vi "FPP-sample-download.vi"() -> ()   [LabVIEW 2016]
panel:
  in  "file path":path
  out "Vp2":dbl[](array[numeric]) format="%.2f"
  out "Time":dbl[](array[numeric]) format="%.2f"
  out "Vp1":dbl[](array[numeric]) format="%.2f"
  out "Id":dbl[](array[numeric]) format="%.2f"
  out "Ig":dbl[](array[numeric]) format="%.2f"
  out "error out":errorcluster
  out "VISA Resource Name out":refnum<visa-resource-name>
  in  "error in (no error)":errorcluster
  in  "VISA resource name in":refnum<visa-resource-name>
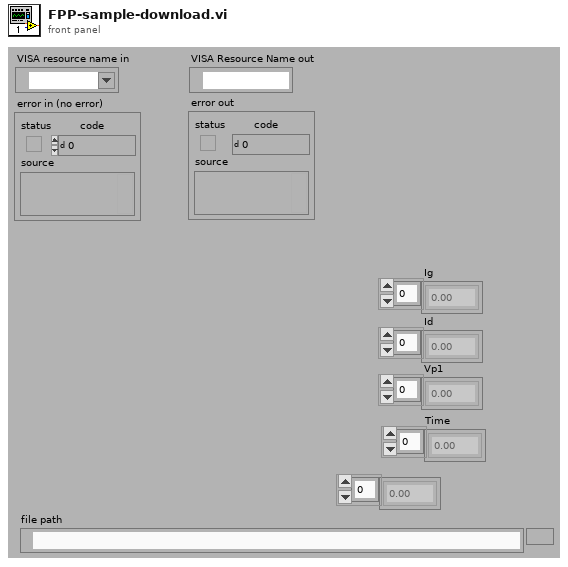
[diagram p1: front panel]
types:
  T1 = enum16{"open", "replace", "create", "open or create", "replace or create", "replace or create with confirmation"}
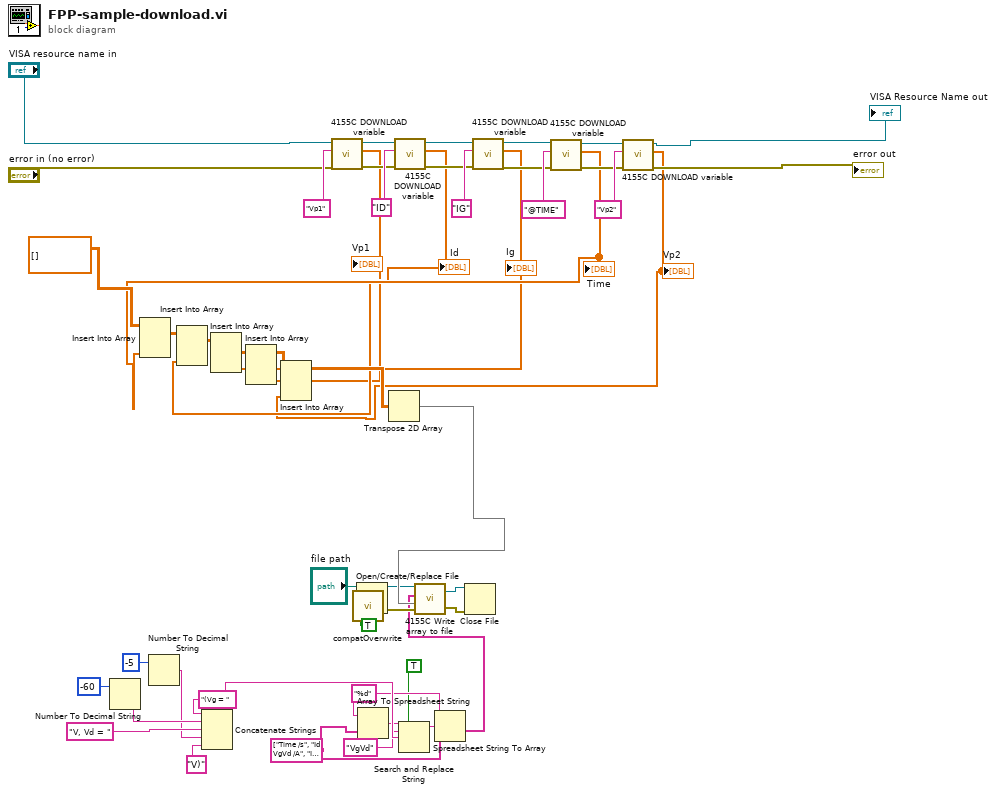
[diagram p0: block diagram]
diagram:
  w12 = string[] ["Time /s", "Id VgVd /A", "Ig VgVd /A", "Vp1 VgVd /V", "Vp2 VgVd /V"] ("Header")
  w16 = "%d" ("format string")
  n1 = Number To Decimal String(number=-60) -> (decimal integer string=w28:string)  [unwired: 1 in]
  n2 = Number To Decimal String(number=-5) -> (decimal integer string=w26:string)  [unwired: 1 in]
  n3 = Concatenate Strings("(Vg = " ("Substring"), w28, "V, Vd = " ("Substring"), w26, "V)" ("Substring")) -> (w24:string)
  n4 = call "4155C DOWNLOAD variable.vi"("error in (no error)"="error in (no error)", "Variable name"="Vp1", "VISA resource name in"="VISA resource name in") -> ("error out"=w49:errorcluster, "Output data"=w3:dbl[], "VISA Resource Name out"=w48:refnum<visa-resource-name>)  [unwired: 2 in]
  "Vp1" <- w3
  n5 = call <vilib>:"compatOverwrite.vi"("overwrite (F)"=TRUE) -> ("overwrite?"=w1:T1)
  n6 = Open/Create/Replace File(file path (use dialog)="file path", operation (0:open)=w1) -> (refnum out=w21:refnum<file>, error out=w22:errorcluster)  [unwired: 4 in, 1 out]
  n7 = Array To Spreadsheet String(array=w12, 3:w16) -> (spreadsheet string=w18:string)  [unwired: 1 in]
  n8 = call "4155C DOWNLOAD variable.vi"("error in (no error)"=w49, "Variable name"="ID", "VISA resource name in"=w48) -> ("error out"=w46:errorcluster, "Output data"=w5:dbl[], "VISA Resource Name out"=w45:refnum<visa-resource-name>)  [unwired: 2 in]
  "Id" <- w5
  n9 = Search and Replace String(replace all?=TRUE ("replace all? (F)"), input string=w18, search string="VgVd", replace string=w24) -> (result string=w14:string)  [unwired: 4 in, 3 out]
  n10 = Spreadsheet String To Array(format string=w16, spreadsheet string=w14, array type (2D Dbl)=w12) -> (array=w13:string[])  [unwired: 1 in]
  n11 = call "4155C DOWNLOAD variable.vi"("error in (no error)"=w46, "Variable name"="IG", "VISA resource name in"=w45) -> ("error out"=w42:errorcluster, "Output data"=w4:dbl[], "VISA Resource Name out"=w43:refnum<visa-resource-name>)  [unwired: 2 in]
  "Ig" <- w4
  n12 = call "4155C DOWNLOAD variable.vi"("error in (no error)"=w42, "Variable name"="@TIME", "VISA resource name in"=w43) -> ("error out"=w39:errorcluster, "Output data"=w6:dbl[], "VISA Resource Name out"=w40:refnum<visa-resource-name>)  [unwired: 2 in]
  "Time" <- w6
  n13 = Insert Into Array(array=dbl[][] [] ("Input Array"), new element=w6) -> (w34:dbl[][])  [unwired: 2 in]
  n14 = Insert Into Array(array=w34, new element=w5) -> (w33:dbl[][])  [unwired: 2 in]
  n15 = Insert Into Array(array=w33, new element=w4) -> (w32:dbl[][])  [unwired: 2 in]
  n16 = Insert Into Array(array=w32, new element=w3) -> (w31:dbl[][])  [unwired: 2 in]
  n17 = call "4155C DOWNLOAD variable.vi"("error in (no error)"=w39, "Variable name"="Vp2", "VISA resource name in"=w40) -> ("error out"=→"error out":errorcluster, "Output data"=w2:dbl[], "VISA Resource Name out"=→"VISA Resource Name out":refnum<visa-resource-name>)  [unwired: 2 in]
  "Vp2" <- w2
  n18 = Insert Into Array(array=w31, new element=w2) -> (w11:dbl[][])  [unwired: 2 in]
  n19 = Transpose 2D Array(2D array=w11) -> (transposed array=w30:dbl[][])
  n20 = call "4155C Write array to file.vi"("Byte Stream File Refnum"=w21, "Header"=w13, "Data Array"=w30, "error in (no error)"=w22) -> ("dup refnum"=w19:refnum<file>, "error out"=w20:errorcluster)  [unwired: 1 in]
  n21 = Close File(refnum=w19, error in=w20) -> ()  [unwired: 2 out]
